vi "readFromXML.vi"(8 "error in (no error)":errorcluster, 10 "XML in":string, 11 "POriginCommands in":refnum<class "POriginCommands.lvclass">) -> (0 "error out":errorcluster, 3 "POriginCommands out":refnum<class "POriginCommands.lvclass">)   [LabVIEW 2014, in "TCSDataDefinitions.lvlib" / "TCSCommand.lvlib" / "POriginCommands.lvlib" / "POriginCommands.lvclass"]
uses:
  POriginCommands.lvclass
  TCSTcsCommand/TCSTcsCommand.lvclass
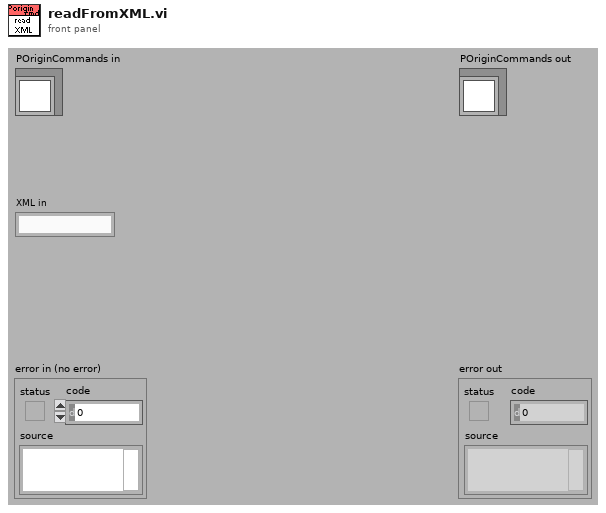
[diagram p1: front panel]
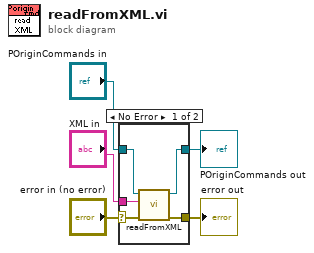
[diagram p0: block diagram]
diagram:
  n1 = case shown="No Error" "error in (no error)" {
    selector: "error in (no error)" -> [w9 w12]
    tunnel: [w8 w12] -> w4
    tunnel: [w6 w11] -> w2
    tunnel: "POriginCommands in" -> [w7 w11]
    tunnel: "XML in" -> [w10 _]
    frame No Error {
      n2 = call-parent "readFromXML.vi"("error in (no error)"=w9, "XMLin"=w10, "TCSTcsCommand in"=w7) -> ("error out"=w8:errorcluster, "TCSTcsCommand out"=w6:refnum<class "POriginCommands.lvclass">)  [unwired: 7 out]
    }
    frame Error {
    }
  }
  "error out" <- w4
  "POriginCommands out" <- w2
